vi "SeCrTs-DI_Read.vi"(8 "error in (no error)":errorcluster, 9 "number of samples per channel":i32, 10 "DI_Task":refnum<k21>, 11 "Data FIFO Ref":T1) -> (0 "error out":errorcluster, 2 "task out":refnum<k21>)   [LabVIEW 2022 SP3]
uses:
  RT Controls/ATF Storage-Data FIFO.ctl
  RT Controls/ATF Storage Haelth.ctl
  <vilib>/DAQmx/read.llb/DAQmx Read (Digital 1D Wfm NChan NSamp).vi
  <vilib>/DAQmx/miscellaneous.llb/DAQmx Fill In Error Info.vi
panel:
  out "overflow?":bool
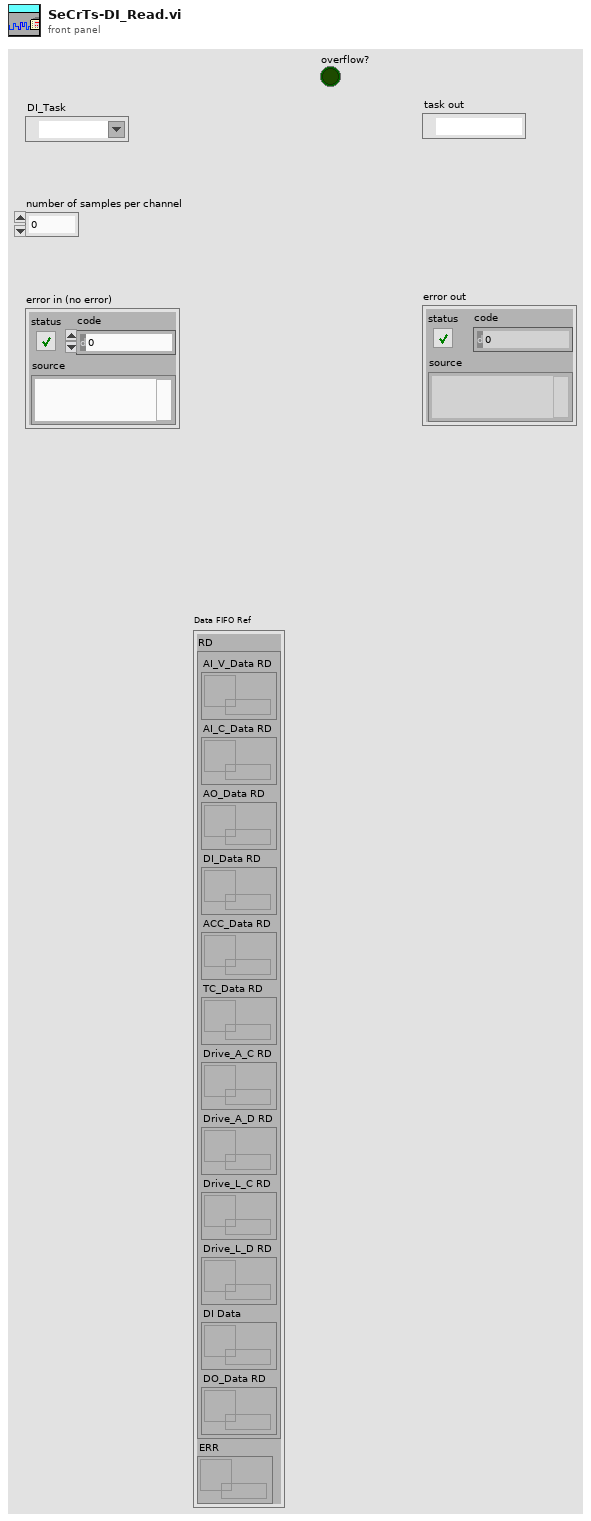
[diagram p1: front panel]
types:
  T1 = typedef "ATF Storage-Data FIFO.ctl" = cluster{"RD":cluster{"AI_V_Data RD":refnum<queue>, "AI_C_Data RD":refnum<queue>, "AO_Data RD":refnum<queue>, "DI_Data RD":refnum<queue>, "ACC_Data RD":refnum<queue>, "TC_Data RD":refnum<queue>, "Drive_A_C RD":refnum<queue>, "Drive_A_D RD":refnum<queue>, "Drive_L_C RD":refnum<queue>, "Drive_L_D RD":refnum<queue>, "DI Data":refnum<queue>, "DO_Data RD":refnum<queue>}, "ERR":refnum<queue>}
  T2 = typedef "ATF Storage Haelth.ctl" = enum16{"AI C", "AI V", "AO", "DI", "DO", "TC", "ACC", "RT Str", "DR A"}
  T3 = enum16{"Init", "Read 'All'", "Read 'n'", "Read '1'", "Write '1'", "Write 'n'", "Write 'All'"}
  T4 = cluster{"Start DAQ":bool, "Stop DAQ":bool, "RT Stop":bool, "RT Exit":bool, "Start Seq":bool}
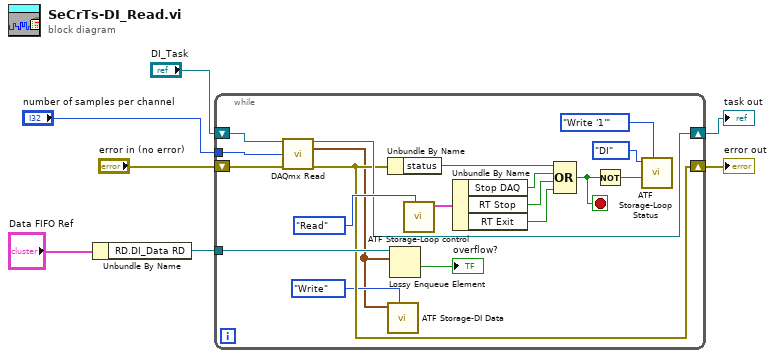
[diagram p0: block diagram]
diagram:
  n1 = Unbundle By Name("Data FIFO Ref") -> ("RD.DI_Data RD"=w1:refnum<queue>)
  n2 = while {
    tunnel: "number of samples per channel" -> [w10]
    tunnel: w1 -> [w14]
    shift-right: [w15] -> w4
    shift-left: "DI_Task" -> [w25]
    shift-right: [w12] -> w3
    shift-left: "error in (no error)" -> [w24]
    stop <- w26 stop-if-true
    n3 = call-poly <vilib>:"DAQmx Read.vi"("task/channels in"=w25, "number of samples per channel"=w10, "error in"=w24) -> ("task out"=w15:refnum<k21>, "data"=w8:digitalwaveform[], "error out"=w12:errorcluster)  [unwired: 10 in]
    n4 = Unbundle By Name(w12) -> ("status"=w23:bool)
    n5 = call "ATF Storage-DI Data.vi"("Enum"=enum16{"Write", "Read"}."Write", "In_DI data"=w8) -> ()  [unwired: 9 in, 1 out]
    n6 = Lossy Enqueue Element(queue=w14, element=w8) -> (overflow?=→"overflow?":bool)  [unwired: 1 in, 3 out]
    n7 = call "ATF Storage-Loop control.vi"("Action"=enum16{"Init", "Write", "Read"}."Read") -> ("Loop Control out"=w18:T4)  [unwired: 9 in, 1 out]
    n8 = Unbundle By Name(w18) -> ("Stop DAQ"=w22:bool, "RT Stop"=w21:bool, "RT Exit"=w20:bool)
    n9 = Compound Arithmetic op=OR(w23, w22, w21, w20) -> (w26:bool)
    n10 = Not(x=w26) -> (.not. x?=w16:bool)
    n11 = call "ATF Storage-Loop Status.vi"("Option"=T3."Write '1'", "Status"=w16, "Loop"=ATF_Storage_Haelth."DI") -> ()  [unwired: 6 in, 3 out]
  }
  "task out" <- w4
  "error out" <- w3
